vi "dlw_gRPC Read.vi"(6 "Worker Alias":string="gRPC Read", 7 "Caller in":refnum<class "Worker.lvclass">, 8 "error in":errorcluster, 10 "Initialization Data":T1, 11 "gRPC Read in":refnum<class "gRPC Read.lvclass">) -> (0 "error out":errorcluster, 3 "gRPC Read out":refnum<class "gRPC Read.lvclass">, 5 "dup Caller out":refnum<class "Worker.lvclass">)   [LabVIEW 2019, in "gRPC Server (template.proto).lvlib" / "gRPC Read.lvclass"]
doc: "This VI dynamically loads the Worker that owns this VI as a subWorker into <b>Caller</b>, and returns the Worker's object containing the Worker's Public Properties. Initialization data that is to be received by this Worker's <Initialize> MHL case can be wired to <b>Initialization Data</b>. The dynamically loaded Worker requires an alias ( <b>Worker Alias</b> ) which must be unique to the Worker it is called from. If a currently loaded subWorker exists with the same Alias, an error will be returned.\n\n<b>Note:</b> This VI can only be used from <b>within</b> a Worker's MHL. To load this Worker from an external LabVIEW application or from TestStand, please use an Asynchronous Launcher VI.\n---"
uses:
  gRPC Read.lvclass
  <vilib>/addons/_Workers/Library/Classes/Worker/Worker.lvclass
  Response Cases.ctl
  Initialization Data.ctl
  <vilib>/addons/_Workers/Library/Case Label.ctl
  <vilib>/addons/_Workers/Library/Workers.lvlib
  <vilib>/gRPC/LabVIEW gRPC Library/Shared/grpcId.ctl
  <vilib>/gRPC/LabVIEW gRPC Library/grpc-lvsupport-release.lvlib
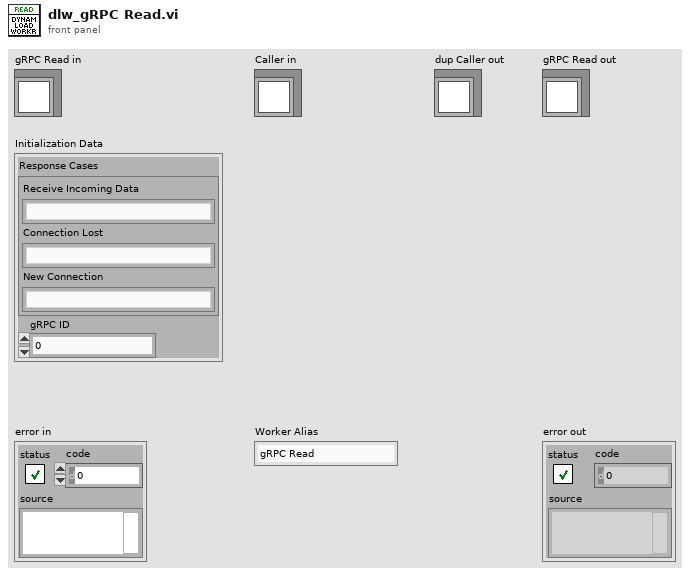
[diagram p1: front panel]
types:
  T1 = typedef "gRPC Server (template.proto).lvlib/gRPC Read.lvclass/Initialization Data.ctl" = cluster{"Response Cases":T2, "gRPC ID":T4}
  T2 = typedef "gRPC Server (template.proto).lvlib/gRPC Read.lvclass/Response Cases.ctl" = cluster{"Receive Incoming Data":T3, "Connection Lost":T3, "New Connection":T3}
  T3 = typedef "Workers.lvlib/Case Label.ctl" = string
  T4 = typedef "grpc-lvsupport-release.lvlib/grpcId.ctl" = u64
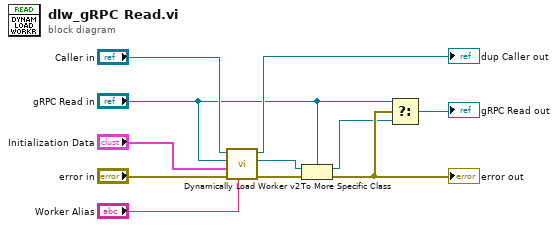
[diagram p0: block diagram]
diagram:
  n1 = call <vilib>:"Dynamically Load Worker v2.vi"("Worker Alias"="Worker Alias", "error in"="error in", "Initialization Data"="Initialization Data", "Worker to Dynamically Load"="gRPC Read in", "Worker"="Caller in") -> ("error out"=w10:errorcluster, "Dynamically Loaded Worker out"=w5:refnum<class "Worker.lvclass">, "dup Worker out"=→"dup Caller out":refnum<class "Worker.lvclass">)  [unwired: 4 in]
  n2 = To More Specific Class(target class="gRPC Read in", reference=w5, error in=w10) -> (specific class reference=w2:refnum<class "gRPC Read.lvclass">, error out=w4:errorcluster)
  "error out" <- w4
  n3 = Select(t="gRPC Read in", s=w4, f=w2) -> (s? t:f=→"gRPC Read out":refnum<class "gRPC Read.lvclass">)
